vi "DrawImageCentre (SubVI).vi"(6 "Axis colour":u32(colorbox)=16711680, 8 "error in (no error)":errorcluster, 11 "Refnum in":T1) -> (0 "error out":errorcluster, 3 "Refnum out":T1)   [LabVIEW 2016]
uses:
  <vilib>/vision/Image Controls.llb/IMAQ Image.ctl
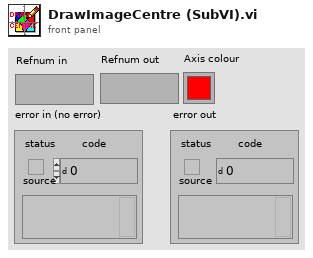
[diagram p1: front panel]
types:
  T1 = typedef "IMAQ Image.ctl" = refnum<image>
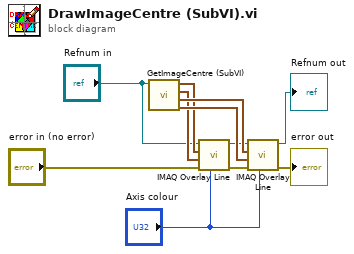
[diagram p0: block diagram]
diagram:
  n1 = call "GetImageCentre (SubVI).vi"("Image in \n(refnum)"="Refnum in") -> ("End y-line"=w9:cluster{"x":i32, dbl}, "Start y-line"=w8:cluster{"x":dbl, dbl}, "End x-line"=w7:cluster{dbl, "y":i32}, "Start x-line"=w6:cluster{dbl, "x":dbl})  [unwired: 4 in, 1 out]
  n2 = call "IMAQ Overlay Line"("Color"="Axis colour", "error in (no error)"="error in (no error)", "End Point"=w7, "Start Point"=w6, "Image"="Refnum in") -> ("error out"=w5:errorcluster, "Image Out"=w4:T1)  [unwired: 5 in]
  n3 = call "IMAQ Overlay Line"("Color"="Axis colour", "error in (no error)"=w5, "End Point"=w9, "Start Point"=w8, "Image"=w4) -> ("error out"=→"error out":errorcluster, "Image Out"=→"Refnum out":T1)  [unwired: 5 in]
